vi "CompileBlockDiagram.vi"(8 "error in":errorcluster, 11 "RasPi Compiler in":refnum<class "RasPi Compiler.lvclass">) -> (0 "error out":errorcluster, 3 "RasPi Compiler out":refnum<class "RasPi Compiler.lvclass">)   [LabVIEW 2014, in "Raspberry Pi Compatible Compiler for LabVIEW.lvlib" / "RasPi Compiler.lvclass"]
uses:
  RasPi Compiler.lvclass
  RasPi Compiler.lvclass/RasPi Compiler.ctl
  Python/PythonConverter_BD/PyConvBD.lvclass
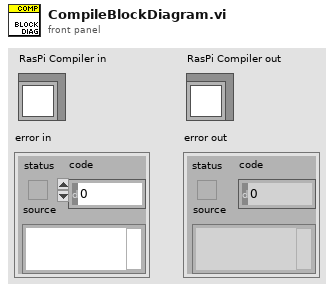
[diagram p1: front panel]
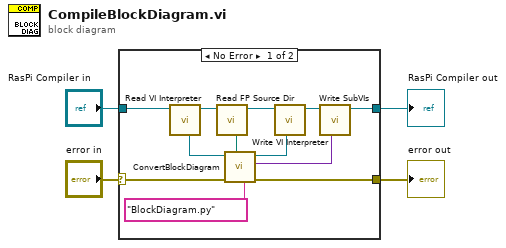
[diagram p0: block diagram]
diagram:
  n1 = case shown="No Error" "error in" {
    selector: "error in" -> [w15 w18]
    tunnel: [w14 w18] -> w3
    tunnel: [w7 w17] -> w1
    tunnel: "RasPi Compiler in" -> [w16 w17]
    frame No Error {
      n2 = call "Read VI Interpreter.vi"("RasPi Compiler in"=w16) -> ("RasPi Compiler out"=w13:refnum<class "RasPi Compiler.lvclass">, "VI Interpreter"=w11:refnum<class "VI Interpreter.lvclass">)  [unwired: 7 in]
      n3 = call "Read FP Source Dir.vi"("RasPi Compiler in"=w13) -> ("RasPi Compiler out"=w12:refnum<class "RasPi Compiler.lvclass">, "FP Source Dir"=w9:path)  [unwired: 7 in]
      n4 = call "ConvertBlockDiagram.vi"("filename"="BlockDiagram.py", "Source Directory"=w9, "error in"=w15, "VI Interpreter"=w11) -> ("error out"=w14:errorcluster, "SubVIs"=w6:variant, "VI Interpreter out"=w10:refnum<class "VI Interpreter.lvclass">)  [unwired: 3 in]
      n5 = call "Write VI Interpreter.vi"("VI Interpreter"=w10, "RasPi Compiler in"=w12) -> ("RasPi Compiler out"=w8:refnum<class "RasPi Compiler.lvclass">)  [unwired: 7 in]
      n6 = call "Write SubVIs.vi"("SubVIs"=w6, "RasPi Compiler in"=w8) -> ("RasPi Compiler out"=w7:refnum<class "RasPi Compiler.lvclass">)  [unwired: 7 in]
    }
    frame Error {
    }
  }
  "error out" <- w3
  "RasPi Compiler out" <- w1
